vi "Servo MSMT LTE Create Evaluations.vi"(8 "error in (no error)":errorcluster, 11 "Servo MSMT in":refnum<class "Servo MSMT.lvclass">) -> (0 "error out":errorcluster, 2 "LTE Evaluations":T1[](array[typedef]) {"Low Limit" format="%#_13g"; "SI Scaling" items=["femto"=-15, "pico"=-12, "nano"=-9, "micro"=-6, "milli"=-3, "percent"=-2, ""=0, "kilo"=3, "mega"=6, "giga"=9, "tera"=12]}, 3 "Servo MSMT out":refnum<class "Servo MSMT.lvclass">)   [LabVIEW 2018, in "Servo MSMT.lvlib" / "Servo MSMT.lvclass"]
uses:
  Servo MSMT.lvclass
  C:/Sequence Automation/Plugins/Measurement Interface.lvlibp/Measurement Interface.lvclass
  Plugins/TestStand API Tools (TSAT).lvlibp/Evaluation Actions/Includes/Controls/TSAT Evaluation.ctl
  Plugins/TestStand API Tools (TSAT).lvlibp/Evaluation Actions/Includes/Controls/TSAT Eval SI Unit Scaling.ctl
  Plugins/TestStand API Tools (TSAT).lvlibp/Evaluation Actions/Includes/Controls/TSAT Evaluation Type.ctl
  Plugins/SeqAuto IEvaluation.lvlibp/SeqAuto IEvaluation.lvclass
  Servo MSMT.lvclass/Servo MSMT.ctl
  Protected Methods/Read DC Pins.vi
  Protected Methods/Read Servo Measurements.vi
  Plugins/SeqAuto Evaluations.lvlibp/LTE Evaluations/LTE_ACP/LTE_ACP.lvclass
  C:/Sequence Automation/Plugins/SeqAuto IEvaluation.lvlibp/SeqAuto IEvaluation.lvclass
  Plugins/SeqAuto Evaluations.lvlibp/LTE Evaluations/LTE_OBW/LTE_OBW.lvclass
  Plugins/SeqAuto Evaluations.lvlibp/LTE Evaluations/LTE_CHP/LTE_CHP.lvclass
  Plugins/SeqAuto Evaluations.lvlibp/LTE Evaluations/LTE_SEM/LTE_SEM.lvclass
  Plugins/SeqAuto Evaluations.lvlibp/Servo/Servo Gain/Servo Gain.lvclass
  Plugins/SeqAuto Evaluations.lvlibp/PA Evaluations/PAE/PAE.lvclass
  Plugins/SeqAuto Evaluations.lvlibp/LTE Evaluations/LTE_ModAcc/LTE_ModAcc.lvclass
  Plugins/SeqAuto Evaluations.lvlibp/DC Evaluations/DC_IDD.lvclass
  Plugins/Measurement Interface.lvlibp/Private Methods/Measurement Name/Read Measurement Name.vi
  Plugins/Measurement Interface.lvlibp/Private Methods/Measurement Parameters/Read Measurement Parameters.vi
  Plugins/String Database.lvlibp/String Database.lvclass
  Plugins/Test Number and Bin Generator.lvlibp/Test Number and Bin Generator/Test Number and Bin Generator.lvclass
  Plugins/TestStand API Tools (TSAT).lvlibp/Evaluation Actions/TSAT Evaluation Actions.lvlib
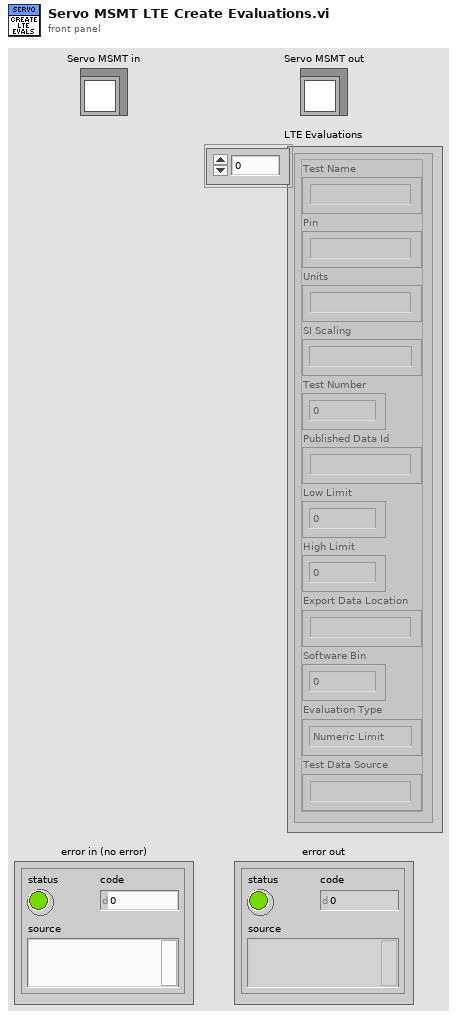
[diagram p1: front panel]
types:
  T1 = typedef "TestStand API Tools (TSAT).lvlibp/TSAT Evaluation Actions.lvlib/TSAT Evaluation.ctl" = cluster{"Test Name":string, "Pin":string, "Units":string, "SI Scaling":T2, "Test Number":i32, "Published Data Id":string, "Low Limit":dbl, "High Limit":dbl, "Export Data Location":string, "Software Bin":i64, "Evaluation Type":T3, "Test Data Source":string}
  T2 = typedef "TestStand API Tools (TSAT).lvlibp/TSAT Evaluation Actions.lvlib/TSAT Eval SI Unit Scaling.ctl" = i16
  T3 = typedef "TestStand API Tools (TSAT).lvlibp/TSAT Evaluation Actions.lvlib/TSAT Evaluation Type.ctl" = enum16{"Numeric Limit", "Pass/Fail", "None"}
  T4 = typedef "Test Number and Bin Generator.lvlibp/Test Number and Bin Generator.lvclass/Session Handle.ctl" = refnum<data-value>
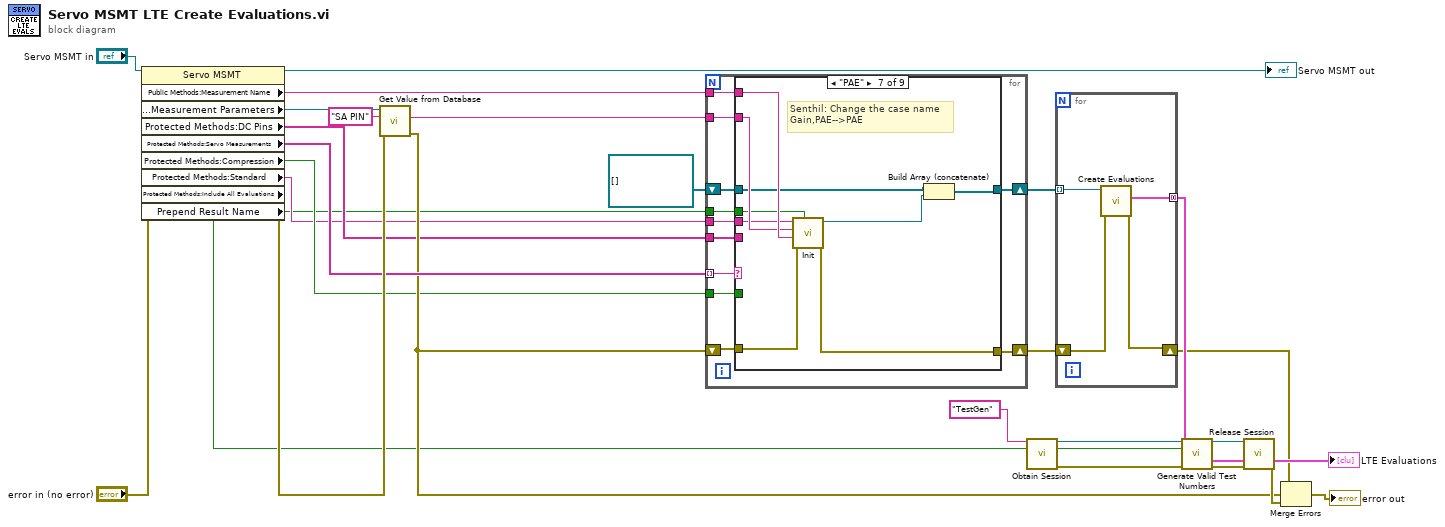
[diagram p0: block diagram]
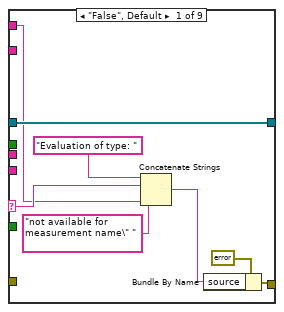
[diagram p2: hidden frame]
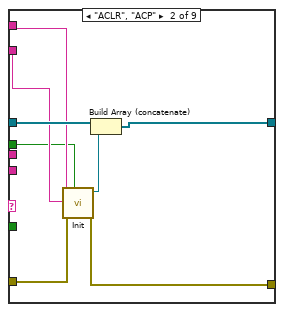
[diagram p3: hidden frame]
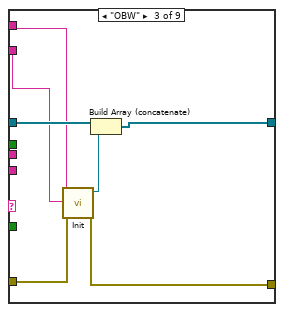
[diagram p4: hidden frame]
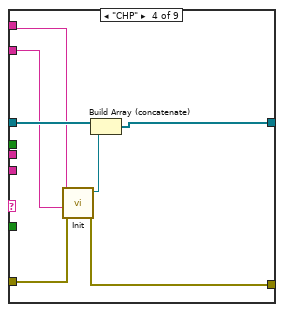
[diagram p5: hidden frame]
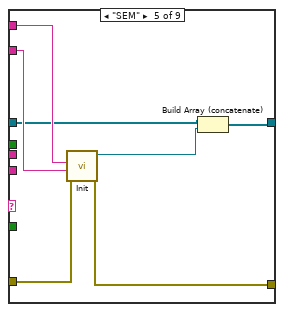
[diagram p6: hidden frame]
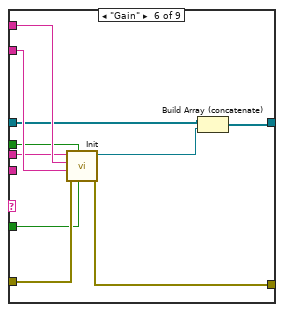
[diagram p7: hidden frame]
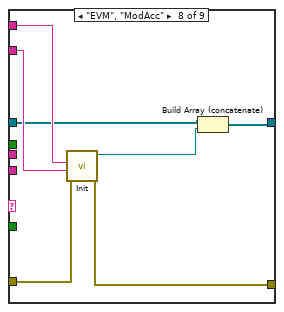
[diagram p8: hidden frame]
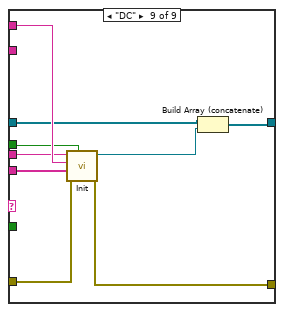
[diagram p9: hidden frame]
diagram:
  n1 = property class="Servo MSMT"(reference="Servo MSMT in", error in="error in (no error)") -> (reference out=→"Servo MSMT out":refnum<class "Servo MSMT.lvclass">, error out=w12:errorcluster, "Public Methods:Measurement Name"=w14:string, "Protected Methods:Measurement Parameters"=w18:refnum<class "String Database.lvclass">, "Protected Methods:DC Pins"=w5:string[], "Protected Methods:Servo Measurements"=w9:string[], "Protected Methods:Compression"=w4:bool, "Protected Methods:Standard"=w3:string, "Protected Methods:Include All Evaluations"=w2:bool, "Prepend Result Name"=w1:bool)
  n2 = call "Get Value from Database.vi"("error in (no error)"=w12, "Entry Name"="SA PIN", "Message in"=w18) -> ("error out"=w8:errorcluster, "Entry Value"=w17:string)  [unwired: 5 in, 2 out]
  n3 = for {
    tunnel: w17 -> [w39]
    tunnel: w14 -> [w38]
    shift-right: [w36] -> w16
    shift-left: refnum<class "SeqAuto IEvaluation.lvclass">[] [] -> [w37]
    tunnel: w9 -> [w35] mode=indexing
    shift-right: [w33] -> w7
    shift-left: w8 -> [w34]
    tunnel: w5 -> [w32]
    tunnel: w3 -> [w31]
    tunnel: w4 -> [w30]
    tunnel: w1 -> [w29]
    n4 = case shown="\"PAE\"" w35 {
      selector: w35 -> [w43 _ _ _ _ _ _ _ _]
      tunnel: w39 -> [_ w49 w56 w63 w75 w85 w94 w101 _]
      tunnel: w38 -> [w41 w50 w57 w64 w76 w86 w95 w102 w111]
      tunnel: [w47 w55 w62 w69 w70 w80 w89 w96 w106] -> w36
      tunnel: w37 -> [w47 w54 w61 w68 w72 w82 w91 w98 w108]
      tunnel: w34 -> [_ w52 w59 w66 w74 w84 w93 w100 w110]
      tunnel: [w45 w51 w58 w65 w73 w83 w92 w99 w109] -> w33
      tunnel: w32 -> [_ _ _ _ _ _ _ _ w105]
      tunnel: w31 -> [_ _ _ _ _ w79 w88 _ w104]
      tunnel: w30 -> [_ _ _ _ _ w78 _ _ _]
      tunnel: w29 -> [_ w48 _ _ _ w77 w87 _ w103]
      frame "False", Default {
        n5 = Concatenate Strings("Evaluation of type: " ("source"), w43, "not available for measurement name\" " ("source"), w41) -> (w40:string)
        n6 = Bundle By Name(cluster=errorcluster {"status"=TRUE, "code"=7777, "source"=""} ("error out"), "source"=w40) -> (w45:errorcluster)
      }
      frame "ACLR", "ACP" {
        n7 = call "Init.vi"("Prepend Result Name"=w48, "error in (no error)"=w52, "SA Pin"=w49, "Measurement Name"=w50) -> ("error out"=w51:errorcluster, "LTE_ACP out"=w53:refnum<class "LTE_ACP.lvclass">)  [unwired: 6 in]
        n8 = Build Array (concatenate)(w54, w53) -> (w55:refnum<class "SeqAuto IEvaluation.lvclass">[])
      }
      frame "OBW" {
        n9 = call "Init.vi"("error in (no error)"=w59, "SA Pin"=w56, "Measurement Name"=w57) -> ("error out"=w58:errorcluster, "LTE_OBW out"=w60:refnum<class "LTE_OBW.lvclass">)  [unwired: 7 in]
        n10 = Build Array (concatenate)(w61, w60) -> (w62:refnum<class "SeqAuto IEvaluation.lvclass">[])
      }
      frame "CHP" {
        n11 = call "Init.vi"("error in (no error)"=w66, "SA Pin"=w63, "Measurement Name"=w64) -> ("error out"=w65:errorcluster, "LTE_CHP out"=w67:refnum<class "LTE_CHP.lvclass">)  [unwired: 7 in]
        n12 = Build Array (concatenate)(w68, w67) -> (w69:refnum<class "SeqAuto IEvaluation.lvclass">[])
      }
      frame "SEM" {
        n13 = call "Init.vi"("error in (no error)"=w74, "SA Pin"=w75, "Measurement Name"=w76) -> ("error out"=w73:errorcluster, "LTE_SEM out"=w71:refnum<class "LTE_SEM.lvclass">)  [unwired: 7 in]
        n14 = Build Array (concatenate)(w72, w71) -> (w70:refnum<class "SeqAuto IEvaluation.lvclass">[])
      }
      frame "Gain" {
        n15 = call "Init.vi"("Compression?"=w78, "Prepend Result Name"=w77, "error in (no error)"=w84, "SA Pin"=w85, "Measurement Name"=w86, "Standard"=w79) -> ("error out"=w83:errorcluster, "Servo Gain out"=w81:refnum<class "Servo Gain.lvclass">)  [unwired: 4 in]
        n16 = Build Array (concatenate)(w82, w81) -> (w80:refnum<class "SeqAuto IEvaluation.lvclass">[])
      }
      frame "PAE" {
        # "Senthil: Change the case name\nGain,PAE-->PAE"
        n17 = call "Init.vi"("Prepend Result Name"=w87, "error in (no error)"=w93, "Measurement Name"=w95, "SA Pin"=w94, "Standard"=w88) -> ("error out"=w92:errorcluster, "PAE out"=w90:refnum<class "PAE.lvclass">)  [unwired: 5 in]
        n18 = Build Array (concatenate)(w91, w90) -> (w89:refnum<class "SeqAuto IEvaluation.lvclass">[])
      }
      frame "EVM", "ModAcc" {
        n19 = call "Init.vi"("error in (no error)"=w100, "SA Pin"=w101, "Measurement Name"=w102) -> ("error out"=w99:errorcluster, "LTE_ModAcc out"=w97:refnum<class "LTE_ModAcc.lvclass">)  [unwired: 7 in]
        n20 = Build Array (concatenate)(w98, w97) -> (w96:refnum<class "SeqAuto IEvaluation.lvclass">[])
      }
      frame "DC" {
        n21 = call "Init.vi"("Prepend Result Name"=w103, "error in (no error)"=w110, "DC Pins"=w105, "Measurement Name"=w111, "Standard"=w104) -> ("error out"=w109:errorcluster, "DC_IDD out"=w107:refnum<class "DC_IDD.lvclass">)  [unwired: 5 in]
        n22 = Build Array (concatenate)(w108, w107) -> (w106:refnum<class "SeqAuto IEvaluation.lvclass">[])
      }
    }
  }
  n23 = call "Obtain Session.vi"("Session  Name ()"="TestGen") -> ("Session Handle"=w24:T4, "error out"=w21:errorcluster)  [unwired: 13 in]
  n24 = for {
    tunnel: w16 -> [w115] mode=indexing
    tunnel: [w114] -> w15 mode=concatenating
    shift-right: [w112] -> w6
    shift-left: w7 -> [w113]
    n25 = call-dynamic "Create Evaluations.vi"("error in (no error)"=w113, "IEvaluation in"=w115) -> ("error out"=w112:errorcluster, "Evaluations Out"=w114:T1[])  [unwired: 7 in, 1 out]
  }
  n26 = call "Generate Valid Test Numbers.vi"("Session Handle in"=w24, "Include All Evaluations?"=w2, "Evaluations In"=w15, "error in (no error)"=w21) -> ("Session Handle out"=w23:T4, "Evaluations Out"=→"LTE Evaluations":T1[], "error out"=w22:errorcluster)  [unwired: 9 in]
  n27 = call "Release Session.vi"("Session Handle"=w23, "error in (no error)"=w22) -> ("error out"=w11:errorcluster)  [unwired: 13 in]
  n28 = Merge Errors(w6, w8, w11) -> (→"error out":errorcluster)
